vi "Measure.vi"(7 "Power Meter reading reference":refnum<vi>, 8 "error in (no error)":errorcluster, 9 "Progress Ref":refnum<vi>, 10 "XY Graph Reference":refnum<vi>, 11 "Harmonics in":refnum<class "Harmonics.lvclass">) -> (0 "error out":errorcluster, 1 "Cal values":cluster{"Name":string, "Value":string}[](array[cluster]), 2 "Results":T1[](array[typedef]), 3 "Harmonics out":refnum<class "Harmonics.lvclass">)   [LabVIEW 2020, in "Harmonics.lvclass"]
uses:
  Harmonics.lvclass
  C:/Sandbox/Git_Sandbox/WiSpry Test Framework source code (LV20)/WiSpry Test Framework/Measurements/Measurement.lvclass
  XML Handler/Controls/Result Cluster.ctl
  Path Control/Paths.ctl
  Harmonics.lvclass/Harmonics.ctl
  Measurement.lvclass/Measurement.ctl
  Instruments/Spectrum Analyzer/Controls/Marker Search.ctl
  Instruments/Spectrum Analyzer/Spectrum Analyzer.lvclass/Spectrum Analyzer.ctl
  Instruments/Spectrum Analyzer/Spectrum Analyzer.lvclass
  Instruments/Signal Generator/Signal Generator.lvclass
  Measurement.lvclass
  Path Control/PathControl.lvclass
  XML Handler/XML Handler.lvclass
  <vilib>/Analysis/NI_AALPro.lvlib
  Instruments/Power Meter/Power Meter.lvclass
panel:
  out "intercept 2":dbl
  out "slope 2":dbl
  out "Best Linear Fit 2":dbl[](array[numeric])
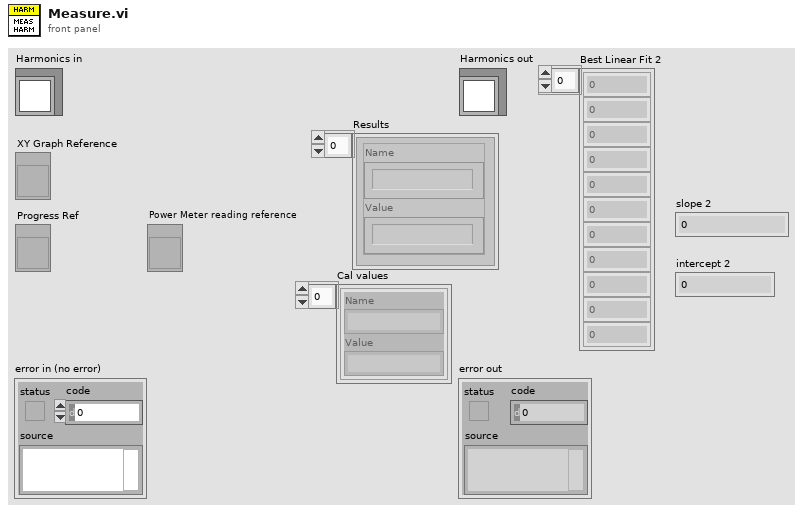
[diagram p1: front panel]
types:
  T1 = typedef "XML Handler.lvclass/Result Cluster.ctl" = cluster{"Name":string, "Value":string}
  T2 = typedef "PathControl.lvclass/Paths.ctl" = enum16{"SigGen 1 -> DUT", "SigGen 2 -> DUT", "SigGen 1 -> PM 1", "SigGen 1 -> PM 2", "DUT -> SA", "DUT -> PM 2", "VSG -> DUT", "SigGen 2 -> PM 1", "SigGen 2 -> PM 2"}
  T3 = typedef "Spectrum Analyzer.lvclass/Marker Search.ctl" = enum16{"Maximum Peak", "Maximum Next", "Maximum Right", "Maximum Left", "Minimum Peak", "Minimum Next", "Minimum Right", "Minimum Left"}
  T4 = typedef "Harmonics.lvclass/Config info.ctl" = cluster{"RBW":dbl, "VBW ":dbl, "Number of Averages":i32, "Average On":bool, "Symbols":i32[], "All Harm":bool, "Loop order":T5, "Power Window":dbl, "Frequency (MHz)":string, "Power (dBm)":string, "PM for power leveling":u8, "Zero span":bool, "Stop level":dbl}
  T5 = typedef "Harmonics.lvclass/Loop order.ctl" = enum16{"Device -> Power -> Frequency", "Device -> Frequency -> Power"}
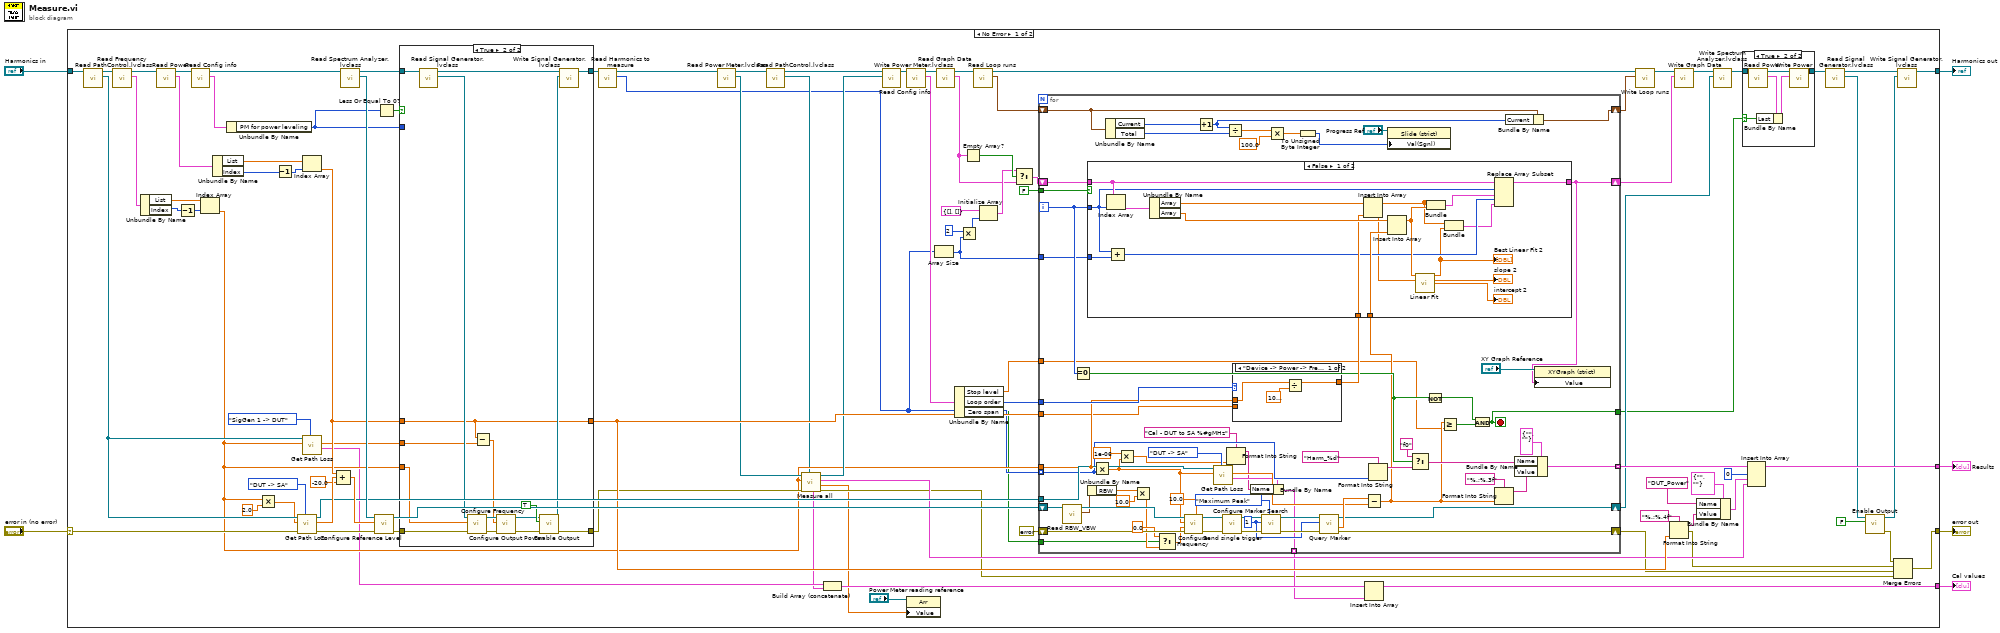
[diagram p0: block diagram]
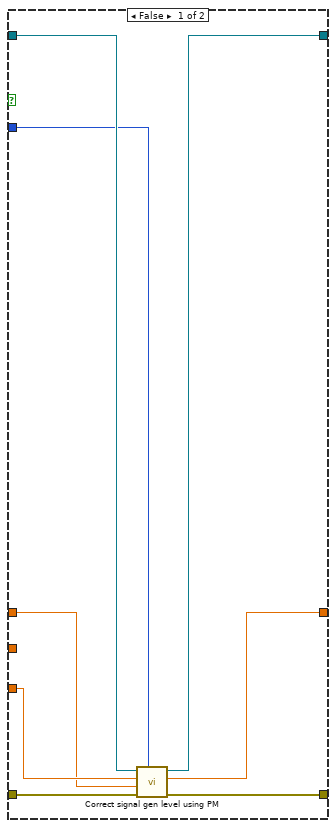
[diagram p3: hidden frame]
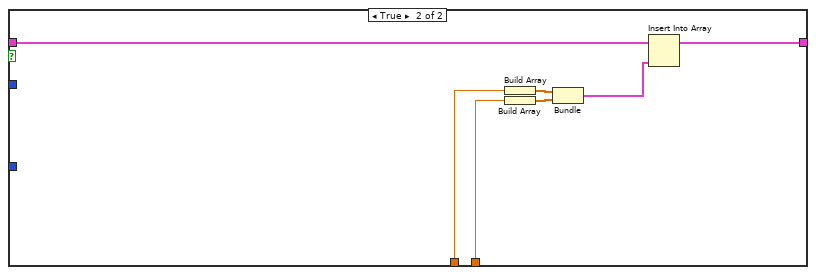
[diagram p4: hidden frame]
diagram:
  n1 = case shown="No Error" "error in (no error)" {
    selector: "error in (no error)" -> [w99 w231]
    tunnel: [w31 w231] -> w5
    tunnel: [w13 w230] -> w3
    tunnel: "Harmonics in" -> [w100 w230]
    tunnel: [w62 _] -> w2
    tunnel: [w37 _] -> w1
    frame No Error {
      n2 = call "Read PathControl.lvclass.vi"("Measurements in"=w100) -> ("PathControl.lvclass"=w69:refnum<class "PathControl.lvclass">, "Measurements out"=w97:refnum<class "Harmonics.lvclass">)  [unwired: 9 in]
      n3 = call "Read Frequency.vi"("Harmonics in"=w97) -> ("Frequency"=w102:cluster{"List":dbl[], "Index":i32, "Last":bool}, "Harmonics out"=w103:refnum<class "Harmonics.lvclass">)  [unwired: 9 in]
      n4 = Unbundle By Name(w102) -> ("List"=w75:dbl[], "Index"=w73:i32)
      n5 = call "Read Power.vi"("Harmonics in"=w103) -> ("Power"=w101:cluster{"List":dbl[], "Index":i32, "Last":bool}, "Harmonics out"=w65:refnum<class "Harmonics.lvclass">)  [unwired: 9 in]
      n6 = Decrement(x=w73) -> (x-1=w72:i32)
      n7 = call "Read Config info.vi"("Harmonics in"=w65) -> ("Config info"=w63:T4, "Harmonics out"=w64:refnum<class "Harmonics.lvclass">)  [unwired: 9 in]
      n8 = Index Array(array=w75, index=w72) -> (element=w47:dbl)
      n9 = Unbundle By Name(w101) -> ("List"=w74:dbl[], "Index"=w71:i32)
      n10 = Unbundle By Name(w63) -> ("PM for power leveling"=w11:u8)
      n11 = Multiply(x=w47, y=2.0) -> (x*y=w46:dbl)
      n12 = Decrement(x=w71) -> (x-1=w70:i32)
      n13 = call "Get Path Loss.vi"("Path"=Paths."DUT -> SA", "error in (no error)"=w99, "Frequency [Hz]"=w46, "PathControl in"=w69) -> ("error out"=w92:errorcluster, "Insertion Loss (dB)"=w96:dbl, "PathControl out"=w88:refnum<class "PathControl.lvclass">)  [unwired: 4 in, 1 out]
      n14 = Index Array(array=w74, index=w70) -> (element=w67:dbl)
      n15 = call "Get Path Loss.vi"("Path"=Paths."SigGen 1 -> DUT", "Frequency [Hz]"=w47, "PathControl in"=w69) -> ("Parameter"=w40:cluster{"Name":string, "Value":string}, "Insertion Loss (dB)"=w66:dbl)  [unwired: 5 in, 2 out]
      n16 = Compound Arithmetic op=ADD(w67, w96, -20.0 ("value")) -> (w93:dbl)
      n17 = call "Read Spectrum Analyzer.lvclass.vi"("Harmonics in"=w64) -> ("Spectrum Analyzer.lvclass"=w94:refnum<class "Spectrum Analyzer.lvclass">, "Harmonics out"=w91:refnum<class "Harmonics.lvclass">)  [unwired: 9 in]
      n18 = call-dynamic "Configure Reference Level.vi"("error in (no error)"=w92, "Reference Level [dBm]"=w93, "Spectrum Analyzer in"=w94) -> ("error out"=w68:errorcluster, "Spectrum Analyzer out"=w89:refnum<class "Spectrum Analyzer.lvclass">)  [unwired: 7 in]
      n19 = Less Or Equal To 0?(x=w11) -> (x <= 0?=w54:bool)
      n20 = case shown="True" w54 {
        tunnel: w91 -> [w115 w134]
        tunnel: [w114 w130] -> w90
        tunnel: [w118 w129] -> w51
        tunnel: w68 -> [w117 w128]
        tunnel: w47 -> [w113 w126]
        tunnel: w67 -> [w112 w119]
        tunnel: w66 -> [_ w121]
        tunnel: [w116 w119] -> w56
        tunnel: w11 -> [w111 _]
        frame False {
          n21 = call "Correct signal gen level using PM.vi"("PM for power leveling"=w111, "error in (no error)"=w117, "Power"=w112, "Frequency"=w113, "Harmonics in"=w115) -> ("error out"=w118:errorcluster, "Power at DUT"=w116:dbl, "Harmonics out"=w114:refnum<class "Harmonics.lvclass">)  [unwired: 4 in]
        }
        frame True {
          n22 = call "Read Signal Generator.lvclass.vi"("Harmonics in"=w134) -> ("Signal Generator.lvclass"=w127:refnum<class "Signal Generator.lvclass">, "Harmonics out"=w132:refnum<class "Harmonics.lvclass">)  [unwired: 9 in]
          n23 = call-dynamic "Configure Frequency.vi"("error in (no error)"=w128, "Frequency [Hz]"=w126, "Signal Generator in"=w127) -> ("error out"=w125:errorcluster, "Signal Generator out"=w124:refnum<class "Signal Generator.lvclass">)  [unwired: 7 in]
          n24 = Subtract(x=w119, y=w121) -> (x-y=w120:dbl)
          n25 = call-dynamic "Configure Output Power.vi"("error in (no error)"=w125, "Output Power [dBm]"=w120, "Signal Generator in"=w124) -> ("error out"=w122:errorcluster, "Signal Generator out"=w123:refnum<class "Signal Generator.lvclass">)  [unwired: 7 in]
          n26 = call-dynamic "Enable Output.vi"("error in (no error)"=w122, "Output Enable (F)"=TRUE, "Signal Generator in"=w123) -> ("error out"=w129:errorcluster, "Signal Generator out"=w133:refnum<class "Signal Generator.lvclass">)  [unwired: 7 in]
          n27 = call "Write Signal Generator.lvclass.vi"("Signal Generator.lvclass"=w133, "Harmonics in"=w132) -> ("Harmonics out"=w130:refnum<class "Harmonics.lvclass">)  [unwired: 9 in]
        }
      }
      n28 = call "Read Harmonics to measure.vi"("Harmonics in"=w90) -> ("Harmonics to measure"=w27:i32[], "Harmonics out"=w50:refnum<class "Harmonics.lvclass">)  [unwired: 9 in]
      n29 = call "Read Power Meter.lvclass.vi"("Harmonics in"=w50) -> ("Power Meter classes"=w52:refnum<class "Power Meter.lvclass">[], "Harmonics out"=w44:refnum<class "Harmonics.lvclass">)  [unwired: 9 in]
      n30 = call "Read PathControl.lvclass.vi"("Measurements in"=w44) -> ("PathControl.lvclass"=w43:refnum<class "PathControl.lvclass">, "Measurements out"=w42:refnum<class "Harmonics.lvclass">)  [unwired: 9 in]
      n31 = call "Measure all.vi"("PathControl in"=w43, "Error In"=w51, "Frequency"=w47, "Power Meter classes"=w52) -> ("Error Out"=w32:errorcluster, "Power readings"=w29:dbl[], "Power results"=w48:T1[], "Power Meter classes"=w53:refnum<class "Power Meter.lvclass">[], "Calibration values"=w39:cluster{"Name":string, "Value":string}[])  [unwired: 3 in]
      n32 = Build Array (concatenate)(w40, w39) -> (w38:cluster{"Name":string, "Value":string}[])
      n33 = call "Write Power Meter.lvclass.vi"("Power Meter classes"=w53, "Harmonics in"=w42) -> ("Harmonics out"=w49:refnum<class "Harmonics.lvclass">)  [unwired: 9 in]
      n34 = property class="Arr"(reference="Power Meter reading reference", "Value"=w29) -> ()  [unwired: 1 in, 2 out]
      n35 = call "Read Config info.vi"("Harmonics in"=w49) -> ("Config info"=w84:T4, "Harmonics out"=w85:refnum<class "Harmonics.lvclass">)  [unwired: 9 in]
      n36 = Array Size(array=w27) -> (size(s)=w24:i32)
      n37 = call "Read Graph Data.vi"("Harmonics in"=w85) -> ("Graph Data"=w19:cluster{"Array":dbl[], "Array":dbl[]}[], "Harmonics out"=w80:refnum<class "Harmonics.lvclass">)  [unwired: 9 in]
      n38 = Unbundle By Name(w84) -> ("Stop level"=w28:dbl, "Loop order"=w83:T5, "Zero span"=w26:bool)
      n39 = Multiply(x=2, y=w24) -> (x*y=w23:i32)
      n40 = Empty Array?(array=w19) -> (empty?=w21:bool)
      n41 = call "Read Loop runs.vi"("Measurements in"=w80) -> ("Loop runs"=w79:cluster{"Current":u32, "Total":u32}, "Measurements out"=w78:refnum<class "Harmonics.lvclass">)  [unwired: 9 in]
      n42 = Initialize Array(cluster{"Array":dbl[], "Array":dbl[]} {"Array"=[], "Array"=[]} ("Cluster"), w23) -> (w20:cluster{"Array":dbl[], "Array":dbl[]}[])
      n43 = Select(t=w20, s=w21, f=w19) -> (s? t:f=w18:cluster{"Array":dbl[], "Array":dbl[]}[])
      n44 = for {
        shift-right: [w178] -> w33
        shift-left: errorcluster {"status"=FALSE, "code"=0, "source"=""} ("error out") -> [w201]
        tunnel: w27 -> [w183] mode=indexing
        tunnel: w47 -> [w174]
        tunnel: w88 -> [w193]
        shift-right: [w177] -> w86
        shift-left: w89 -> [w200]
        tunnel: [w176] -> w87 mode=indexing
        shift-right: [w158] -> w81
        shift-left: w18 -> [w171]
        tunnel: w83 -> [w175]
        tunnel: w56 -> [w173]
        shift-right: [w167] -> w76
        shift-left: w79 -> [w168]
        tunnel: FALSE ("empty?") -> [w159]
        tunnel: [w152] -> w36 mode=indexing
        tunnel: w28 -> [w142]
        tunnel: w24 -> [w141]
        tunnel: w26 -> [w137]
        tunnel: [w135] -> w15
        i -> [w157]
        stop <- w135 stop-if-true
        w186 = u32 1 ("Marker Number (1)")
        n45 = call "Read RBW_VBW.vi"("Spectrum Analyzer in"=w200) -> ("RBW/VBW"=w198:cluster{"RBW":dbl, "VBW":dbl}, "Spectrum Analyzer out"=w199:refnum<class "Spectrum Analyzer.lvclass">)  [unwired: 9 in]
        n46 = Equal To 0?(x=w157) -> (x = 0?=w146:bool)
        n47 = Unbundle By Name(w198) -> ("RBW"=w197:dbl)
        n48 = Multiply(x=w174, y=w183) -> (x*y=w150:dbl)
        n49 = Unbundle By Name(w168) -> ("Current"=w169:u32, "Total"=w165:u32)
        n50 = Multiply(x=1e-06, y=w150) -> (x*y=w148:dbl)
        n51 = Multiply(x=w197, y=10.0) -> (x*y=w139:dbl)
        n52 = Select(t=0.0 ("y"), s=w137, f=w139) -> (s? t:f=w138:dbl)
        n53 = call-dynamic "Configure Frequency.vi"("Sweep time (ms)"=10.0, "error in (no error)"=w201, "Span/Stop Frequency [Hz]"=w138, "Center/Start Frequency [Hz]"=w150, "Spectrum Analyzer in"=w199) -> ("error out"=w195:errorcluster, "Spectrum Analyzer out"=w194:refnum<class "Spectrum Analyzer.lvclass">)  [unwired: 5 in]
        n54 = Increment(x=w169) -> (x+1=w166:u32)
        n55 = call "Get Path Loss.vi"("Path"=Paths."DUT -> SA", "Frequency [Hz]"=w150, "PathControl in"=w193) -> ("Parameter"=w153:cluster{"Name":string, "Value":string}, "Insertion Loss (dB)"=w179:dbl)  [unwired: 5 in, 2 out]
        n56 = call-dynamic "Send single trigger.vi"("error in (no error)"=w195, "Spectrum Analyzer in"=w194) -> ("error out"=w191:errorcluster, "Spectrum Analyzer out"=w190:refnum<class "Spectrum Analyzer.lvclass">)  [unwired: 8 in]
        n57 = Divide(x=w166, y=w165) -> (x/y=w164:dbl)
        n58 = Format Into String(format string="Cal - DUT to SA %#gMHz" ("Name"), w148) -> (resulting string=w147:string)  [unwired: 2 in, 1 out]
        n59 = case shown="\"Device -> Power -> Frequency\", Default" w175 {
          tunnel: w174 -> [w228 _]
          tunnel: w173 -> [_ w229]
          tunnel: [w227 w229] -> w172
          frame "Device -> Power -> Frequency", Default {
            n60 = Divide(x=w228, y=1000000.0) -> (x/y=w227:dbl)
          }
          frame "Device -> Frequency -> Power" {
          }
        }
        n61 = Bundle By Name(cluster=w153, "Name"=w147) -> (w152:cluster{"Name":string, "Value":string})
        n62 = call-dynamic "Configure Marker Search.vi"("Marker Search (Max Peak)"=Marker_Search."Maximum Peak", "error in (no error)"=w191, "Marker Number (1)"=w186, "Spectrum Analyzer in"=w190) -> ("error out"=w188:errorcluster, "Spectrum Analyzer out"=w187:refnum<class "Spectrum Analyzer.lvclass">)  [unwired: 6 in]
        n63 = Multiply(x=w164, y=100.0) -> (x*y=w162:dbl)
        n64 = To Unsigned Byte Integer(number=w162) -> (unsigned 8bit integer=w160:u8)
        n65 = call-dynamic "Query Marker.vi"("error in (no error)"=w188, "Marker Number (1)"=w186, "Spectrum Analyzer in"=w187) -> ("error out"=w178:errorcluster, "Marker Level"=w180:dbl, "Spectrum Analyzer out"=w177:refnum<class "Spectrum Analyzer.lvclass">)  [unwired: 5 in, 1 out]
        n66 = Subtract(x=w180, y=w179) -> (x-y=w144:dbl)
        n67 = case shown="False" w159 {
          tunnel: w144 -> [w215 w224]
          tunnel: w172 -> [w214 w225]
          tunnel: w171 -> [w213 w221]
          tunnel: w157 -> [w206 _]
          tunnel: [w211 w219] -> w158
          tunnel: w141 -> [w207 _]
          frame False {
            n68 = Index Array(array=w213, index=w206) -> (element=w218:cluster{"Array":dbl[], "Array":dbl[]})
            n69 = Add(x=w206, y=w207) -> (x+y=w205:i32)
            n70 = Unbundle By Name(w218) -> ("Array"=w217:dbl[], "Array"=w216:dbl[])
            n71 = Insert Into Array(array=w217, new element=w214) -> (w204:dbl[])  [unwired: 1 in]
            n72 = Insert Into Array(array=w216, new element=w215) -> (w208:dbl[])  [unwired: 1 in]
            n73 = call <vilib>:"Linear Fit.vi"("Y"=w208, "X"=w204) -> ("Best Linear Fit"=w203:dbl[], "slope"=→"slope 2":dbl, "intercept"=→"intercept 2":dbl)  [unwired: 9 in, 2 out]
            "Best Linear Fit 2" <- w203
            n74 = Bundle("Array"=w204, "Array"=w208) -> (w212:cluster{"Array":dbl[], "Array":dbl[]})  [unwired: 1 in]
            n75 = Bundle("Array"=w204, "Best Linear Fit"=w203) -> (w202:cluster{"Array":dbl[], "Best Linear Fit":dbl[]})  [unwired: 1 in]
            n76 = Replace Array Subset(array=w213, new element #1=w212, index #1=w206, new element #2=w202, index #2=w205) -> (w211:cluster{"Array":dbl[], "Array":dbl[]}[])
          }
          frame True {
            n77 = Build Array(w225) -> (w223:dbl[])
            n78 = Build Array(w224) -> (w222:dbl[])
            n79 = Bundle(w223, w222) -> (w220:cluster{dbl[], dbl[]})  [unwired: 1 in]
            n80 = Insert Into Array(array=w221, new element=w220) -> (w219:cluster{"Array":dbl[], "Array":dbl[]}[])  [unwired: 1 in]
          }
        }
        n81 = Format Into String(format string="Harm_%d", w183) -> (resulting string=w156:string)  [unwired: 2 in, 1 out]
        n82 = property class="Slide (strict)"(reference="Progress Ref", "Val(Sgnl)"=w160) -> ()  [unwired: 1 in, 2 out]
        n83 = Select(t="f0", s=w146, f=w156) -> (s? t:f=w155:string)
        n84 = Not(x=w146) -> (.not. x?=w145:bool)
        n85 = Greater Or Equal?(x=w144, y=w142) -> (x >= y?=w143:bool)
        n86 = And(x=w145, y=w143) -> (x .and. y?=w135:bool)
        n87 = Format Into String(format string="%.;%.3f", w144) -> (resulting string=w182:string)  [unwired: 2 in, 1 out]
        n88 = Bundle By Name(cluster=w168, "Current"=w166) -> (w167:cluster{"Current":u32, "Total":u32})
        n89 = Bundle By Name(cluster=T1 {"Name"="", "Value"=""} ("Result Cluster"), "Name"=w155, "Value"=w182) -> (w176:T1)
        n90 = property class="XYGraph (strict)"(reference="XY Graph Reference", "Value"=w158) -> ()  [unwired: 1 in, 2 out]
      }
      n91 = Insert Into Array(array=w38, new element=w36) -> (w37:cluster{"Name":string, "Value":string}[])  [unwired: 1 in]
      n92 = call "Write Loop runs.vi"("Loop runs"=w76, "Measurements in"=w78) -> ("Measurements out"=w77:refnum<class "Harmonics.lvclass">)  [unwired: 9 in]
      n93 = Format Into String(format string="%.;%.4f", w56) -> (resulting string=w57:string, error out=w34:errorcluster)  [unwired: 2 in]
      n94 = call "Write Graph Data.vi"("Graph Data"=w81, "Harmonics in"=w77) -> ("Harmonics out"=w82:refnum<class "Harmonics.lvclass">)  [unwired: 9 in]
      n95 = Bundle By Name(cluster=T1 {"Name"="", "Value"=""} ("new element/subarray"), "Name"="DUT_Power", "Value"=w57) -> (w55:T1)
      n96 = call "Write Spectrum Analyzer.lvclass.vi"("Spectrum Analyzer.lvclass"=w86, "Harmonics in"=w82) -> ("Harmonics out"=w16:refnum<class "Harmonics.lvclass">)  [unwired: 9 in]
      n97 = case shown="True" w15 {
        selector: w15 -> [_ w106]
        tunnel: [w104 w109] -> w12
        tunnel: w16 -> [w104 w108]
        frame False {
        }
        frame True {
          n98 = call "Read Power.vi"("Harmonics in"=w108) -> ("Power"=w107:cluster{"List":dbl[], "Index":i32, "Last":bool}, "Harmonics out"=w105:refnum<class "Harmonics.lvclass">)  [unwired: 9 in]
          n99 = Bundle By Name(cluster=w107, "Last"=w106) -> (w110:cluster{"List":dbl[], "Index":i32, "Last":bool})
          n100 = call "Write Power.vi"("Power"=w110, "Harmonics in"=w105) -> ("Harmonics out"=w109:refnum<class "Harmonics.lvclass">)  [unwired: 9 in]
        }
      }
      n101 = Insert Into Array(array=w87, index=0, new element #1=w55, new element #2=w48) -> (w62:T1[])
      n102 = call "Read Signal Generator.lvclass.vi"("Harmonics in"=w12) -> ("Signal Generator.lvclass"=w7:refnum<class "Signal Generator.lvclass">, "Harmonics out"=w14:refnum<class "Harmonics.lvclass">)  [unwired: 9 in]
      n103 = call-dynamic "Enable Output.vi"("Output Enable (F)"=FALSE, "Signal Generator in"=w7) -> ("error out"=w9:errorcluster, "Signal Generator out"=w8:refnum<class "Signal Generator.lvclass">)  [unwired: 8 in]
      n104 = Merge Errors(w9, w34, w33, w32) -> (w31:errorcluster)
      n105 = call "Write Signal Generator.lvclass.vi"("Signal Generator.lvclass"=w8, "Harmonics in"=w14) -> ("Harmonics out"=w13:refnum<class "Harmonics.lvclass">)  [unwired: 9 in]
    }
    frame Error {
    }
  }
  "error out" <- w5
  "Harmonics out" <- w3
  "Results" <- w2
  "Cal values" <- w1
